vi "Event Handle Loop_Add Page.vi"(8 "error in (no error)":errorcluster, 10 "Pag Attribute":T1, 11 "QTab Class in":refnum<class "QTab Class.lvclass">) -> (0 "error out":errorcluster, 3 "QTab Class out":refnum<class "QTab Class.lvclass">)   [LabVIEW 2020, in "QTab.lvlib" / "QTab Class.lvclass"]
uses:
  QTab Class.lvclass
  Pag Attribute.ctl
  QTab Class.lvclass/QTab Class.ctl
  Command.ctl
  QMenu Class/Button Attribute.ctl
  QMenu Class/QMenu Class.lvclass
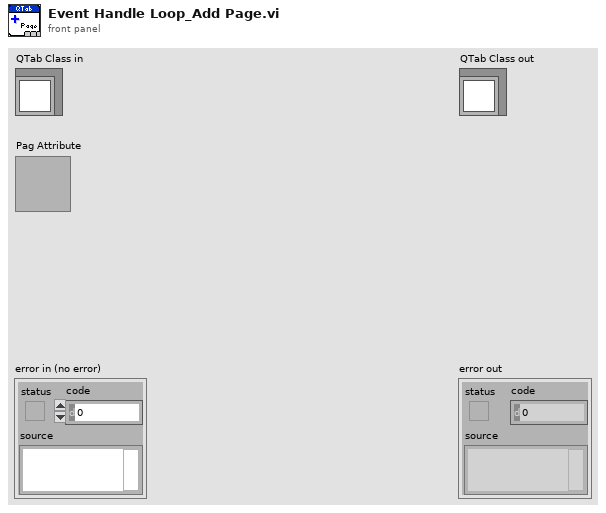
[diagram p1: front panel]
types:
  T1 = typedef "QTab.lvlib/QTab Class.lvclass/Pag Attribute.ctl" = cluster{"VI Refnum":refnum<vi>, "Page Name":string, "Closeable":bool, "Draggable":bool, "Pop-Out":bool}
  T2 = typedef "QTab.lvlib/QTab Class.lvclass/Command.ctl" = enum16{"Startup", "Add Page", "Close All Page", "Set Page Attribute", "Pop-out", "Merage", "Insert", "Stop"}
  T3 = typedef "QTab.lvlib/QMenu Class.lvclass/Button Attribute.ctl" = cluster{"Label":string, "Button Text":string, "Closable":bool, "Draggable":bool}
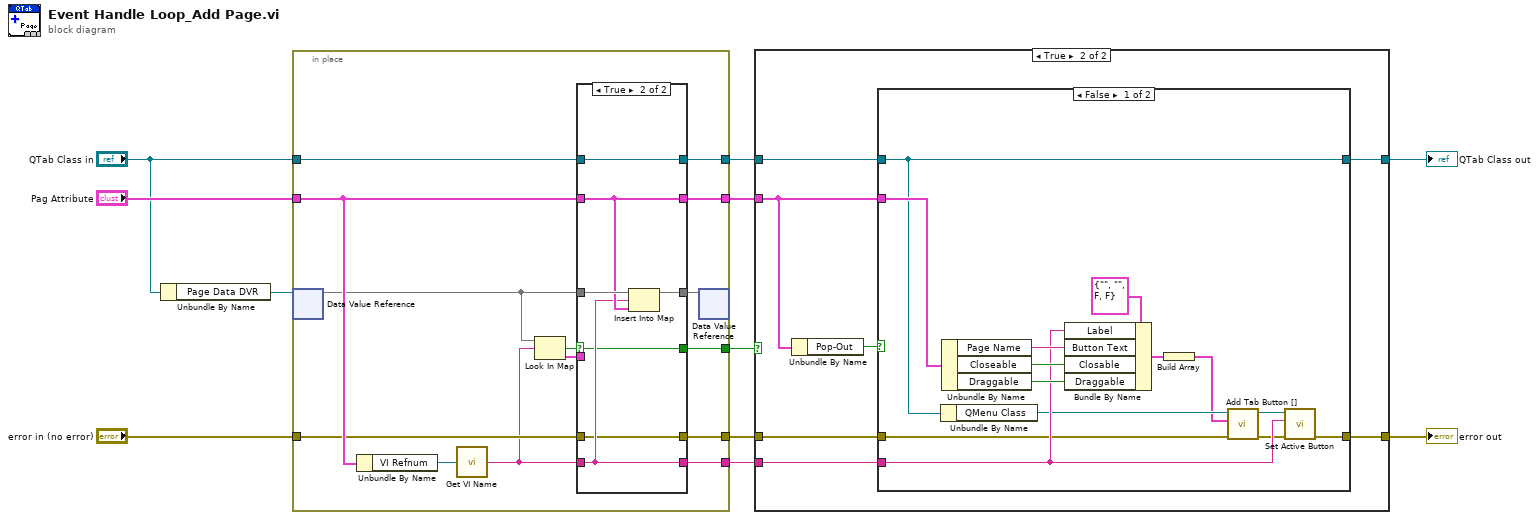
[diagram p0: block diagram]
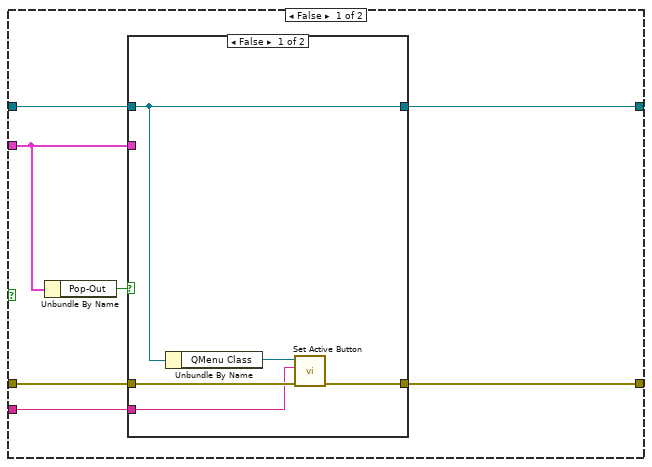
[diagram p2: hidden frame]
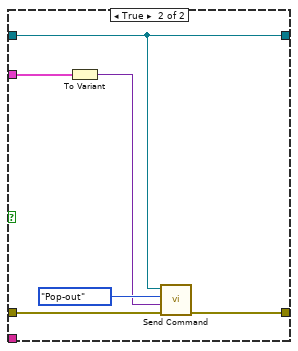
[diagram p3: hidden frame]
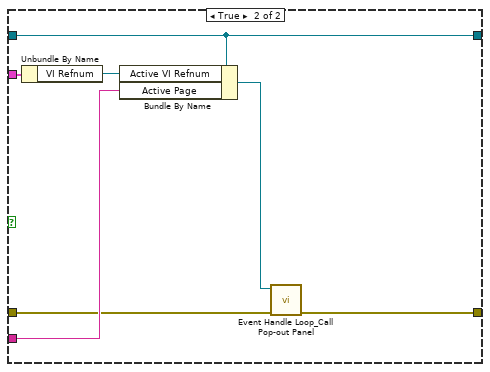
[diagram p4: hidden frame]
diagram:
  n1 = Unbundle By Name("QTab Class in") -> ("Page Data DVR"=w9:refnum<data-value>)
  n2 = in-place {
    in-place-border: "Pag Attribute" -> [w24]
    in-place-border: "QTab Class in" -> [w22]
    in-place-border: [w21] -> w3
    in-place-border: "error in (no error)" -> [w14]
    in-place-border: [w15] -> w7
    in-place-border: [w20] -> w6
    in-place-border: [w17] -> w5
    in-place-border: [w16] -> w4
    n3 = in-place-dvr #1(w9) -> (w19:map{string, T1})  [unwired: 1 out]
    n4 = Unbundle By Name(w24) -> ("VI Refnum"=w12:refnum<vi>)
    n5 = call "Get VI Name.vi"("VI Refnum"=w12) -> ("VI Name"=w13:string)
    n6 = Look In Map(map=w19, key=w13) -> (key not found?=w25:bool, value=w23:T1)  [unwired: 1 in]
    n7 = case shown="True" w25 {
      selector: w25 -> [w27 w33]
      tunnel: w24 -> [_ w36]
      tunnel: w23 -> [w30 _]
      tunnel: w22 -> [w29 w38]
      tunnel: [w29 w38] -> w21
      tunnel: [w30 w36] -> w20
      tunnel: w19 -> [w31 w37]
      tunnel: w13 -> [w28 w34]
      tunnel: [w31 w35] -> w18
      tunnel: [w28 w34] -> w17
      tunnel: [w27 w33] -> w16
      tunnel: w14 -> [w26 w32]
      tunnel: [w26 w32] -> w15
      frame False {
      }
      frame True {
        n8 = Insert Into Map(map in=w37, key=w34, value=w36) -> (map out=w35:map{string, T1})  [unwired: 2 out]
      }
    }
    n9 = in-place-dvr #1(w18) -> ()  [unwired: 2 out]
  }
  n10 = case shown="True" w4 {
    tunnel: w7 -> [w45 w60]
    tunnel: w6 -> [w41 w59]
    tunnel: [w40 w62] -> w1
    tunnel: w5 -> [w39 w63]
    tunnel: w3 -> [w43 w61]
    tunnel: [w42 w57] -> w2
    frame False {
      n11 = Unbundle By Name(w41) -> ("Pop-Out"=w44:bool)
      n12 = case shown="False" w44 {
        tunnel: w45 -> [w50 w56]
        tunnel: w43 -> [w47 w54]
        tunnel: [w47 w54] -> w42
        tunnel: w41 -> [_ w52]
        tunnel: [w49 w55] -> w40
        tunnel: w39 -> [w46 _]
        frame False {
          n13 = Unbundle By Name(w47) -> ("QMenu Class"=w48:refnum<class "QMenu Class.lvclass">)
          n14 = call "Set Active Button.vi"("error in (no error)"=w50, "Label"=w46, "QMenu Class in"=w48) -> ("error out"=w49:errorcluster)  [unwired: 7 in, 1 out]
        }
        frame True {
          n15 = To Variant(anything=w52) -> (Variant=w51:variant)
          n16 = call "Send Command.vi"("error in (no error)"=w56, "Data"=w51, "Command"=Command."Pop-out", "QTab Class in"=w54) -> ("error out"=w55:errorcluster)  [unwired: 6 in, 1 out]
        }
      }
    }
    frame True {
      n17 = Unbundle By Name(w59) -> ("Pop-Out"=w58:bool)
      n18 = case shown="False" w58 {
        tunnel: w63 -> [w73 w80]
        tunnel: [w72 w84] -> w62
        tunnel: w61 -> [w64 w81]
        tunnel: w60 -> [w71 w78]
        tunnel: w59 -> [w65 w83]
        tunnel: [w64 w81] -> w57
        frame False {
          n19 = Unbundle By Name(w64) -> ("QMenu Class"=w68:refnum<class "QMenu Class.lvclass">)
          n20 = Unbundle By Name(w65) -> ("Page Name"=w76:string, "Closeable"=w75:bool, "Draggable"=w74:bool)
          n21 = Bundle By Name(cluster=T3 {"Label"="", "Button Text"="", "Closable"=FALSE, "Draggable"=FALSE} ("Button Attribute"), "Label"=w73, "Button Text"=w76, "Closable"=w75, "Draggable"=w74) -> (w67:T3)
          n22 = Build Array(w67) -> (w66:T3[])
          n23 = call "Add Tab Button [].vi"("error in (no error)"=w71, "Button Attribute []"=w66, "QMenu Class in"=w68) -> ("error out"=w70:errorcluster, "QMenu Class out"=w69:refnum<class "QMenu Class.lvclass">)  [unwired: 7 in]
          n24 = call "Set Active Button.vi"("error in (no error)"=w70, "Label"=w73, "QMenu Class in"=w69) -> ("error out"=w72:errorcluster)  [unwired: 7 in, 1 out]
        }
        frame True {
          n25 = Unbundle By Name(w83) -> ("VI Refnum"=w82:refnum<vi>)
          n26 = Bundle By Name(cluster=w81, "Active VI Refnum"=w82, "Active Page"=w80) -> (w79:refnum<class "QTab Class.lvclass">)
          n27 = call "Event Handle Loop_Call Pop-out Panel.vi"("error in (no error)"=w78, "QTab Class in"=w79) -> ("error out"=w84:errorcluster)  [unwired: 8 in, 1 out]
        }
      }
    }
  }
  "error out" <- w1
  "QTab Class out" <- w2
